vi "Transform command.vi"(1 "Command in":string) -> (0 "Comamnd out":string)   [LabVIEW 2015]
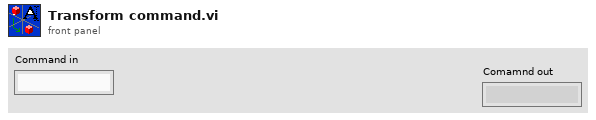
[diagram p1: front panel]
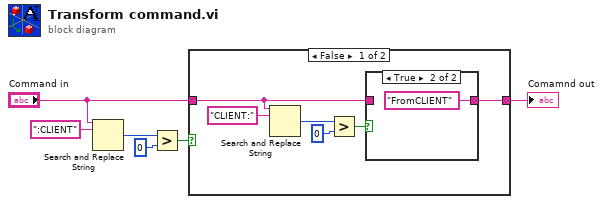
[diagram p0: block diagram]
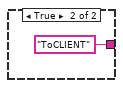
[diagram p3: hidden frame]
diagram:
  n1 = Search and Replace String(input string="Command in", search string=":CLIENT") -> (number of replacements=w5:i32)  [unwired: 6 in, 3 out]
  n2 = Greater?(x=w5, y=0) -> (0:w3:bool)
  n3 = case shown="False" w3 {
    tunnel: "Command in" -> [w8 _]
    tunnel: [w9 "ToCLIENT" ("Command in")] -> w1
    frame False {
      n4 = Search and Replace String(input string=w8, search string="CLIENT:") -> (number of replacements=w11:i32)  [unwired: 6 in, 3 out]
      n5 = Greater?(x=w11, y=0) -> (0:w10:bool)
      n6 = case shown="True" w10 {
        tunnel: [w13 "FromCLIENT" ("Command in")] -> w9
        tunnel: w8 -> [w13 _]
        frame False {
        }
        frame True {
        }
      }
    }
    frame True {
    }
  }
  "Comamnd out" <- w1
